vi "GetPicture.vi"() -> ()   [LabVIEW 2010]
panel:
  in  "GetPicture":bool
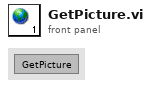
[diagram p1: front panel]
diagram:
